vi "Washing_FGV.vi"(7 "Command":enum16{"SET", "GET"}(ring), 8 "error in (no error)":errorcluster, 11 "Elased_Time(s)":dbl) -> (0 "error out":errorcluster, 3 "Elased_Time(s)_OUT":dbl)   [LabVIEW 2017]
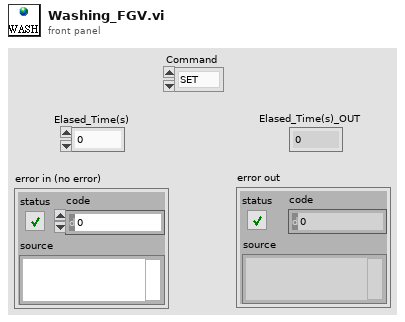
[diagram p1: front panel]
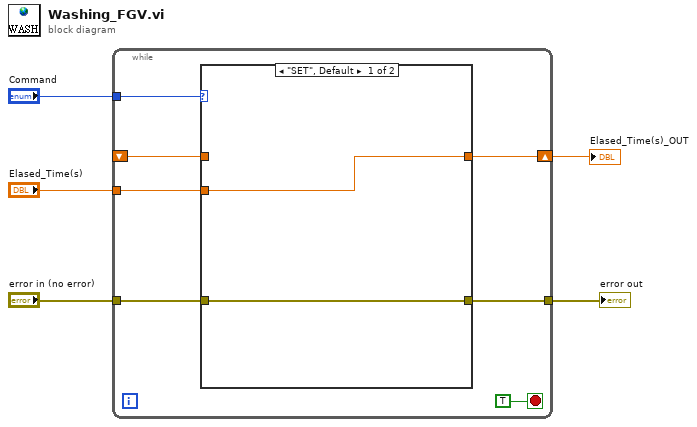
[diagram p0: block diagram]
diagram:
  n1 = while {
    tunnel: "Command" -> [w11]
    shift-right: [w10] -> w3
    shift-left: _ -> [w8]
    tunnel: "Elased_Time(s)" -> [w9]
    tunnel: [w7] -> w2
    tunnel: "error in (no error)" -> [w6]
    stop <- TRUE stop-if-true
    n2 = case shown="\"SET\", Default" w11 {
      tunnel: [w14 w16] -> w10
      tunnel: w9 -> [w14 _]
      tunnel: w8 -> [_ w16]
      tunnel: [w13 w15] -> w7
      tunnel: w6 -> [w13 w15]
      frame "SET", Default {
      }
      frame "GET" {
      }
    }
  }
  "Elased_Time(s)_OUT" <- w3
  "error out" <- w2
